vi "Vision (SubVI).vi"(11 "stop":bool) -> (0 "error out":errorcluster, 1 "GREEN?":bool, 2 "RED?":bool, 3 "Iteration Duration":i64)   [LabVIEW 2017]
uses:
  <vilib>/Platform/TimedLoop/XDataNode/timing_clust.ctl
  <vilib>/Platform/TimedLoop/XDataNode/nitl_modes.ctl
  <vilib>/Platform/TimedLoop/XDataNode/wakeup.ctl
  <vilib>/Platform/TimedLoop/XDataNode/XDataNode.xnode
  <vilib>/Platform/TimedLoop/XDataNode/XDNodeRunTimeDep.lvlib
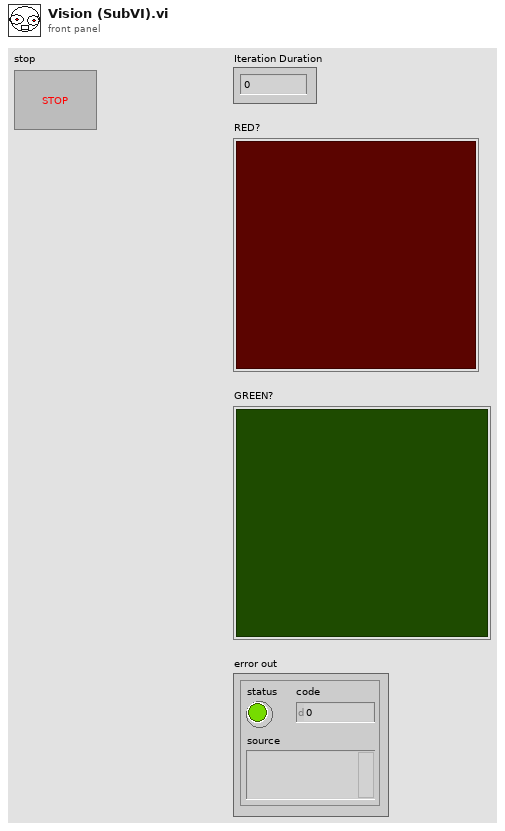
[diagram p1: front panel]
types:
  T1 = typedef "XDNodeRunTimeDep.lvlib/timing_clust.ctl" = cluster{"Expected End [f-1]":u64, "Actual End [f-1]":u64, "Finished Late? [f-1]":bool, "Expected End [i-1]":u64, "Actual End [i-1]":u64, "Finished Late? [i-1]":bool, "Expected Start [i]":u64, "Actual Start [i]":u64, "Expected Start [f]":u64, "Actual Start [f]":u64, "Source Name":string, "Structure Name":string, "Period":i64, "Deadline":i64, "Offset":i64, "Start":i64, "Priority":i32, "Timeout":i32, "Mode":T2, "Wakeup Reason":T3, "Error":errorcluster, "Source Type":string, "Secondary Source Type":string, "Global End Time":u64, "Global Start Time":u64, "Frame Duration":u64, "Iteration Duration":u64, "Assigned CPU":i32, "I/O Scan Engine Mode":u32}
  T2 = typedef "XDNodeRunTimeDep.lvlib/nitl_modes.ctl" = enum32{"No Change", "Process missed periods, maintain original phase", "Discard missed periods, maintain original phase", "Process missed periods, ignore original phase", "Discard missed periods, ignore original phase"}
  T3 = typedef "XDNodeRunTimeDep.lvlib/wakeup.ctl" = enum32{"Normal", "Aborted", "Asynchronous wakeup", "Timing source error", "Timed loop error", "Timeout"}
  T4 = typedef "IMAQ Image.ctl" = refnum<image>
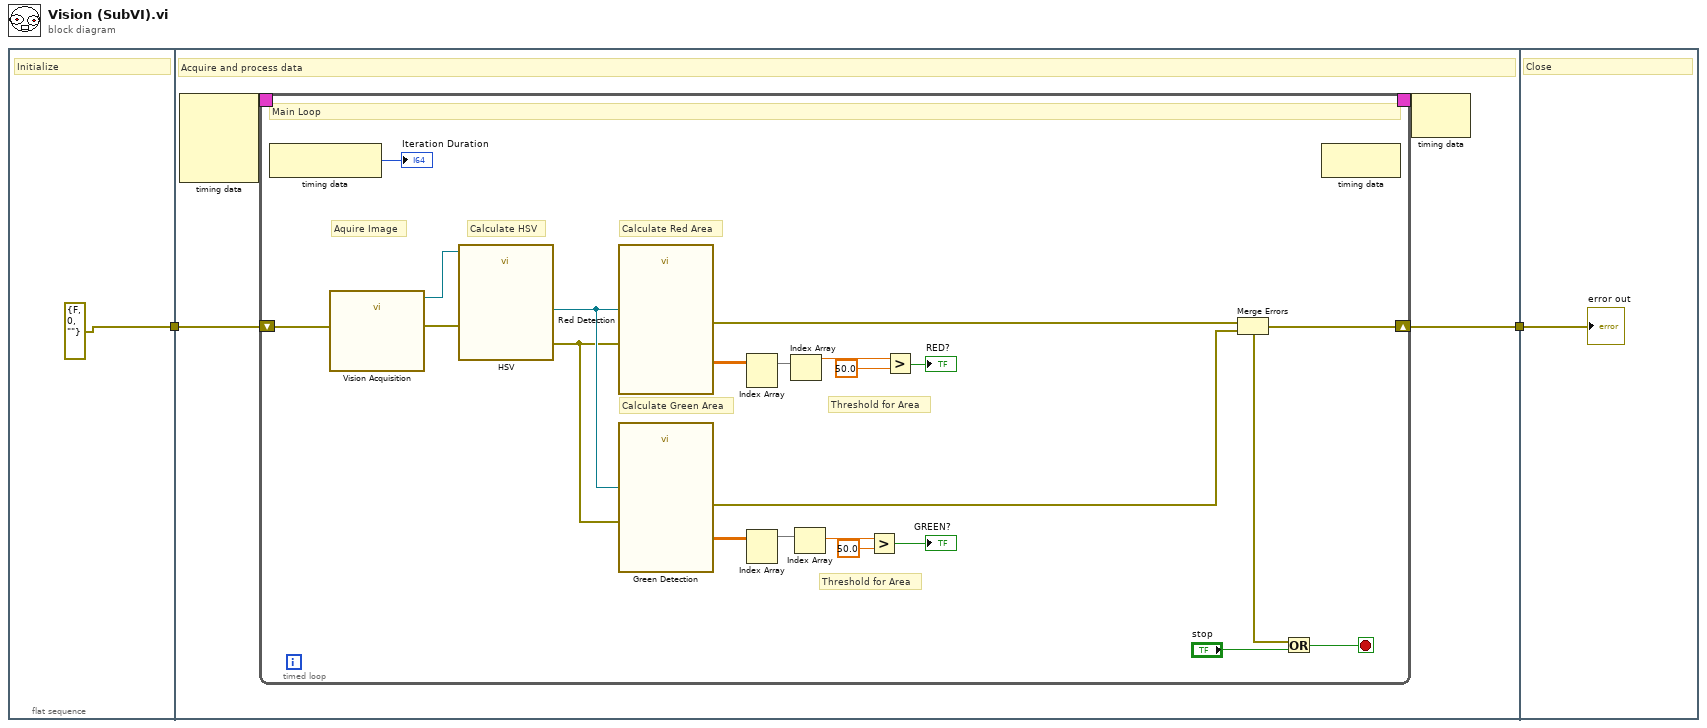
[diagram p0: block diagram]
diagram:
  n1 = flat-sequence {
    tunnel: [errorcluster {"status"=FALSE, "code"=0, "source"=""} ("error in (no error)")] -> w2
    tunnel: w2 -> [w7]
    tunnel: [w6] -> w1
    tunnel: w1 -> [w34]
    frame #0 {
      # "Initialize"
    }
    frame #1 {
      # "Acquire and process data"
      n2 = node-c288() -> (w5:T1)  [unwired: 4 in]
      n3 = timed-loop {
        shift-right: [w9] -> w6
        shift-left: w7 -> [w27]
        timing: w5 -> [_]
        timing-out: [_] -> w4
        stop <- w8 stop-if-true
        # "Calculate Green Area"
        # "Calculate Red Area"
        # "Calculate HSV"
        # "Aquire Image"
        # "Threshold for Area"
        # "Threshold for Area"
        # "Main Loop"
        n4 = node-c288() -> (→"Iteration Duration":i64)  [unwired: 1 in]
        n5 = call "Vision Acquisition"("error in"=w27) -> ("Image Out"=w28:T4, "error out"=w26:errorcluster)  [unwired: 24 in, 1 out]
        n6 = call "HSV"("Image In"=w28, "error in"=w26) -> ("Image Out"=w14:T4, "error out"=w13:errorcluster)  [unwired: 24 in]
        n7 = call "Red Detection"("Image In"=w14, "error in"=w13) -> ("Particle Measurements (Pixels) (Particle Analysis 1)"=w21:dbl[][], "error out"=w11:errorcluster)  [unwired: 23 in, 1 out]
        n8 = call "Green Detection"("Image In"=w14, "error in"=w13) -> ("Particle Measurements (Pixels) (Particle Analysis 1)"=w17:dbl[][], "error out"=w10:errorcluster)  [unwired: 23 in, 1 out]
        n9 = Index Array(array=w21) -> (element=w15:dbl[])  [unwired: 2 in]
        n10 = Index Array(array=w17) -> (element=w20:dbl[])  [unwired: 2 in]
        n11 = Index Array(array=w15) -> (element=w25:dbl)  [unwired: 1 in]
        n12 = Index Array(array=w20) -> (element=w19:dbl)  [unwired: 1 in]
        n13 = Greater?(x=w19, y=50.0) -> (0:→"GREEN?":bool)
        n14 = Greater?(x=w25, y=50.0) -> (0:→"RED?":bool)
        n15 = Merge Errors(w11, w10) -> (w9:errorcluster)
        n16 = Or(x=w9, y="stop") -> (x .or. y?=w8:bool)
        n17 = node-c288() -> ()  [unwired: 1 in, 1 out]
      }
      n18 = node-c288(w4) -> ()  [unwired: 1 out]
    }
    frame #2 {
      # "Close"
      "error out" <- w34
    }
  }
